vi "File Filter by Extension.vi"(8 "error in (no error)":errorcluster, 10 "Extension to filter for":string="tdms", 11 "selected path":path) -> (0 "error out":errorcluster, 1 "Array of Matching full path names":string[](array[string]), 2 "Array of Matching filenames":string[](array[string]), 3 "path out":path)   [LabVIEW 2016]
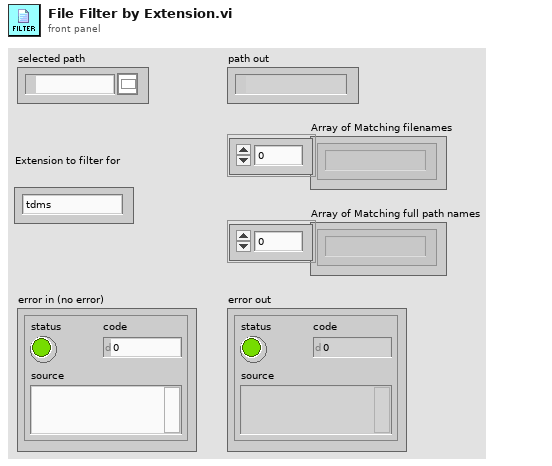
[diagram p1: front panel]
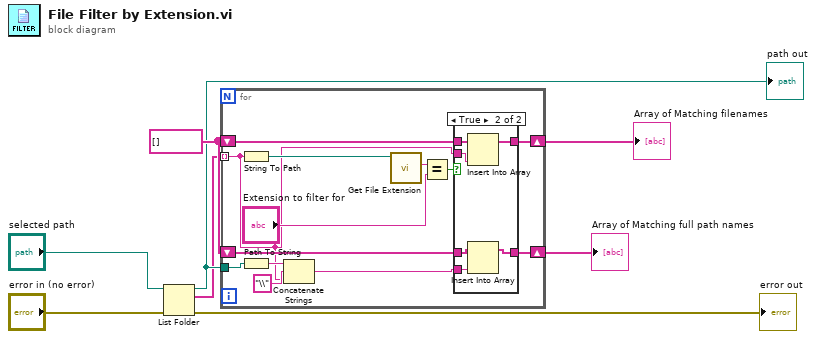
[diagram p0: block diagram]
diagram:
  w6 = string[] [] ("filenames")
  n1 = List Folder(path="selected path", error in="error in (no error)") -> (path out=w3:path, filenames=w2:string[], error out=→"error out":errorcluster)  [unwired: 2 in, 1 out]
  "path out" <- w3
  n2 = for {
    tunnel: w2 -> [w11] mode=indexing
    shift-right: [w17] -> w4
    shift-left: w6 -> [w16]
    tunnel: w3 -> [w15]
    shift-right: [w10] -> w7
    shift-left: w6 -> [w9]
    n3 = String To Path(string=w11) -> (path=w21:path)
    n4 = Path To String(path=w15) -> (string=w14:string)
    n5 = Concatenate Strings(w14, "\\" ("string"), w11) -> (w12:string)
    n6 = call <vilib>:"Get File Extension.vi"("file"=w21) -> ("lowercase file extension"=w20:string)  [unwired: 6 in, 4 out]
    n7 = Equal?(x=w20, y="Extension to filter for") -> (x = y?=w18:bool)
    n8 = case shown="True" w18 {
      tunnel: [w23 w28] -> w17
      tunnel: w16 -> [w23 w29]
      tunnel: w12 -> [_ w27]
      tunnel: w11 -> [_ w26]
      tunnel: [w22 w25] -> w10
      tunnel: w9 -> [w22 w24]
      frame False {
      }
      frame True {
        n9 = Insert Into Array(array=w24, new element=w26) -> (w25:string[])  [unwired: 1 in]
        n10 = Insert Into Array(array=w29, new element=w27) -> (w28:string[])  [unwired: 1 in]
      }
    }
  }
  "Array of Matching filenames" <- w7
  "Array of Matching full path names" <- w4
